vi "BRig_RT__Case_Exp__recordAnalogInput__PortC__fifo.vi"(0 "input_dataAnalog":u16[][](array[numeric]), 2 "input_iOccurence":u16, 3 "resetOccurrence":bool, 4 "input_dataCurrent":u16[](array[numeric]), 6 "input_iState_start":T1, 7 "input_fifo_hdl":refnum<k33>, 8 "input_iState_end":T1, 9 "input_fifo_error":errorcluster, 10 "input_AI1":i16, 12 "input_AI0":i16) -> (11 "output_fifo_error":errorcluster, 13 "output_fifo_hdl":refnum<k33>, 14 "output_dataAnalog":u16[][](array[numeric]), 16 "output_iOccurrence":u16)   [LabVIEW 2014]
uses:
  myRIO_BRig_RT__Case_Exp_stateList.ctl
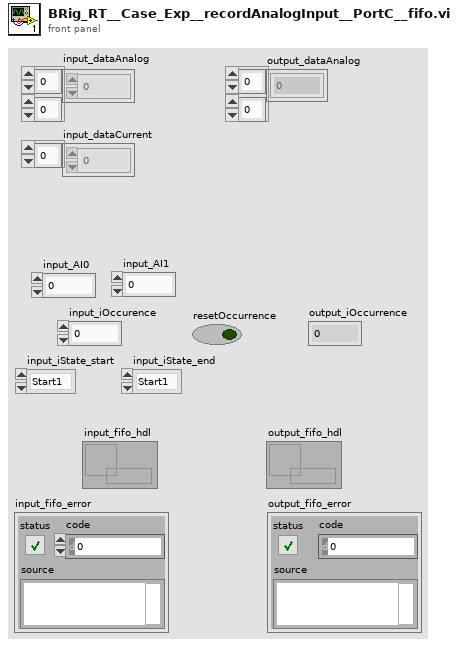
[diagram p1: front panel]
types:
  T1 = typedef "myRIO_BRig_RT__Case_Exp_stateList.ctl" = enum16{"Start1", "Start2", "Start3", "saveSettings1", "saveSettings2", "saveSettings3", "saveSettings4", "saveSettings_LC_ENL_l1", "saveSettings_LC_ENL_l2", "saveSettings_LC_Cue_l1", "saveSettings_LC_Cue_l2", "saveSettings6_LC_l1_Other", "SaveSettings6_LC_l2_Other", "setSettings_Audio", "setSettings_Laser", "initBlock_pre", "initBlock", "initBlock2", "initBlock_post", "initTrial_pre", "initTrial", "initTrial2", "initTrial3", "initTrial4", "initTrial_LC_ENL1", "initTrial_LC_Cue1", "initTrial_LC_Cue1_2", "initTrial_LC_Sel", "initTrial_post", "ENL1_pre", "ENL1", "ENL1_post", "ENL1Penalty_pre", "ENL1Penalty", "ENL2_pre", "ENL2", "ENL2Penalty_pre", "ENL2Penalty", "Cue1_pre", "Cue1", "Cue1_post", "Cue1Penalty_pre", "Cue1Penalty", "Cue2_pre", "Cue2", "Cue2Penalty_pre", "Cue2Penalty", "Selection_pre", "Selection", "Select_post", "SelectReward_pre", "SelectReward", "SelectRewardPost_pre", "SelectRewardPost", "SelectWrong_pre", "SelectWrong", "SelectWrong_post", "SelectTimeout_pre", "SelectTimeout", "SelectTimeout_post", "endTrial_pre", "endTrial1", "endTrial2", "endTrial3", "endTrial_post", "endBlock_pre", "endBlock", "endBlock_post", "endExp", "commConnect", "commUpload_pre", "commUpload_dataBlock", "commUpload_dataCurrent", "commUpload_dataExp", "commUpload_dataLC", "commUpload_dataTrial", "commUpload_post", "saveData_pre", "saveData_dataBlock", "saveData_dataCurrent", "saveData_dataExp", "saveData_dataLC", "saveData_dataTrial", "saveData_post", "empty_endBlock1", "empty_endBlock2", "empty_endTrial1", "empty_endTrial2", "empty_endTrial3", "empty_endTrial4", "empty_endTrial5", "dummyState", "dummyState_endBlock", "FreeReward_pre", "FreeReward", "FreeRewardPost_pre", "FreeRewardPost"}
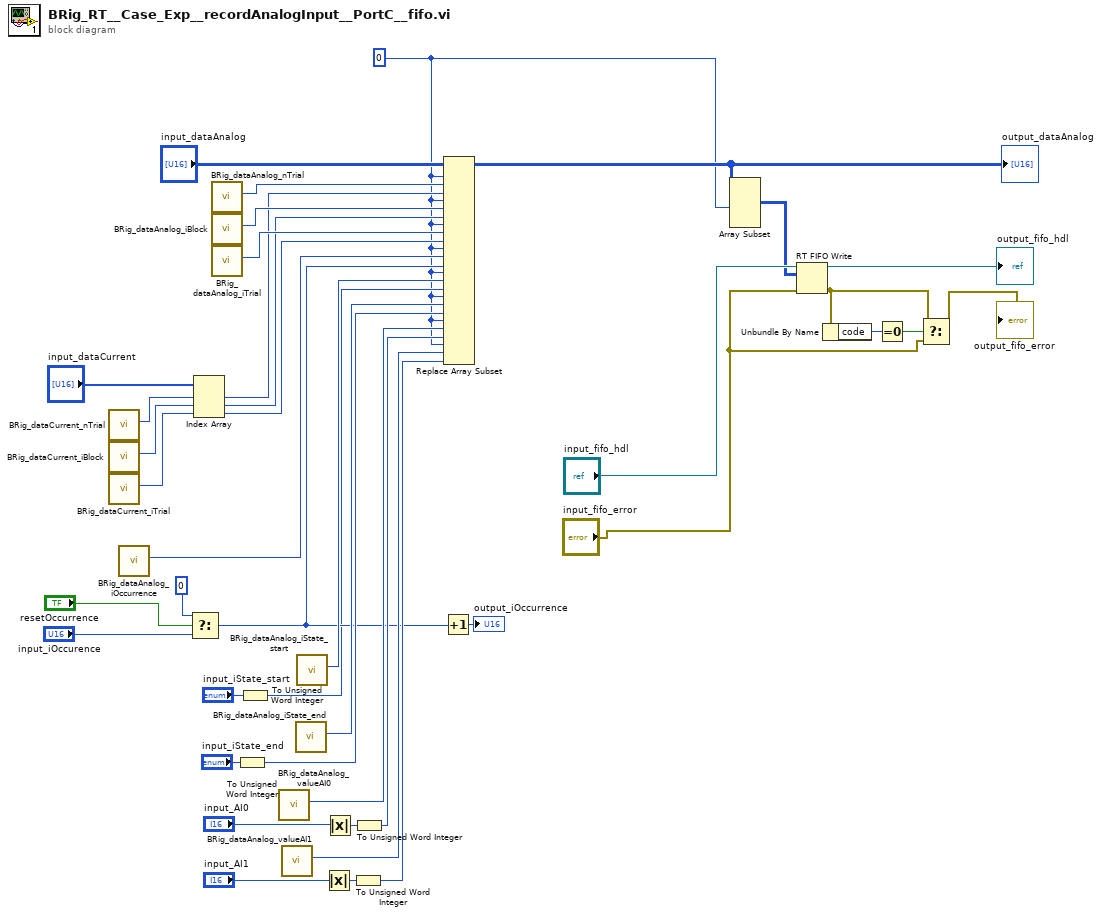
[diagram p0: block diagram]
diagram:
  w9 = 0
  n1 = call "BRig_dataCurrent_nTrial.vi"() -> ("output_nTrial"=w37:i32)  [unwired: 11 in]
  n2 = call "BRig_dataCurrent_iBlock.vi"() -> ("output_iBlock"=w36:i32)  [unwired: 11 in]
  n3 = call "BRig_dataCurrent_iTrial.vi"() -> ("output_iTrial"=w35:i32)  [unwired: 11 in]
  n4 = call "BRig_dataAnalog_iOccurrence.vi"() -> ("output_iOccurrence"=w28:i32)  [unwired: 11 in]
  n5 = Select(t=u16 0, s="resetOccurrence", f="input_iOccurence") -> (s? t:f=w19:u16)
  n6 = Index Array(array="input_dataCurrent", index #1=w37, index #2=w36, index #3=w35) -> (element #1=w13:u16, element #2=w14:u16, element #3=w12:u16)
  n7 = call "BRig_dataAnalog_nTrial.vi"() -> ("output_nTrial"=w34:i32)  [unwired: 11 in]
  n8 = call "BRig_dataAnalog_iBlock.vi"() -> ("output_iBlock"=w33:i32)  [unwired: 11 in]
  n9 = call "BRig_dataAnalog_iTrial.vi"() -> ("output_iTrial"=w32:i32)  [unwired: 11 in]
  n10 = To Unsigned Word Integer(number="input_iState_end") -> (unsigned 16bit integer=w27:u16)
  n11 = To Unsigned Word Integer(number="input_iState_start") -> (unsigned 16bit integer=w10:u16)
  n12 = call "BRig_dataAnalog_valueAI0.vi"() -> ("output_valueAI0"=w26:i32)  [unwired: 11 in]
  n13 = call "BRig_dataAnalog_valueAI1.vi"() -> ("output_valueAI1"=w25:i32)  [unwired: 11 in]
  n14 = call "BRig_dataAnalog_iState_end.vi"() -> ("output_iState_end"=w29:i32)  [unwired: 11 in]
  n15 = call "BRig_dataAnalog_iState_start.vi"() -> ("output_iState_start"=w30:i32)  [unwired: 11 in]
  n16 = Absolute Value(x="input_AI1") -> (abs(x)=w39:i16)
  n17 = Absolute Value(x="input_AI0") -> (abs(x)=w40:i16)
  n18 = To Unsigned Word Integer(number=w39) -> (unsigned 16bit integer=w23:u16)
  n19 = To Unsigned Word Integer(number=w40) -> (unsigned 16bit integer=w24:u16)
  n20 = Increment(x=w19) -> (x+1=→"output_iOccurrence":u16)
  n21 = Replace Array Subset(array="input_dataAnalog", new element #1=w13, index (row) #1=w9, index (col) #1=w34, new element #2=w14, index (row) #2=w9, index (col) #2=w33, new element #3=w12, index (row) #3=w9, index (col) #3=w32, new element #4=w19, index (row) #4=w9, index (col) #4=w28, new element #5=w10, index (row) #5=w9, index (col) #5=w30, new element #6=w27, index (row) #6=w9, index (col) #6=w29, new element #7=w24, index (row) #7=w9, index (col) #7=w26, new element #8=w23, index (row) #8=w9, index (col) #8=w25) -> (w11:u16[][])
  "output_dataAnalog" <- w11
  n22 = Array Subset(array=w11, length (row)=w9) -> (w2:u16[][])  [unwired: 3 in]
  n23 = RT FIFO Write(0:"input_fifo_hdl", 1:w2, 3:"input_fifo_error") -> (8:→"output_fifo_hdl":refnum<k33>, 11:w1:errorcluster)  [unwired: 2 in, 2 out]
  n24 = Unbundle By Name(w1) -> ("code"=w4:i32)
  n25 = Equal To 0?(x=w4) -> (x = 0?=w3:bool)
  n26 = Select(t=w1, s=w3, f="input_fifo_error") -> (s? t:f=→"output_fifo_error":errorcluster)
